vi "Load Budget.vi"(8 "error in (no error)":errorcluster, 11 "Budgetizer in":refnum<class "Budgetizer.lvclass">) -> (0 "error out":errorcluster, 3 "Budgetizer out":refnum<class "Budgetizer.lvclass">)   [LabVIEW 2018, in "Budgetizer.lvclass"]
uses:
  Budgetizer.lvclass
  Budgetizer.lvclass/Budgetizer.ctl
  database/Database.lvclass
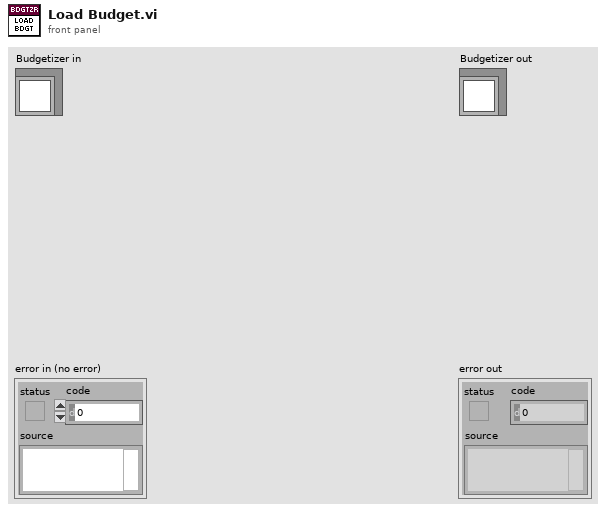
[diagram p1: front panel]
types:
  T1 = enum16{"January", "February", "March", "April", "May", "June", "July", "August", "September", "October", "November", "December"}
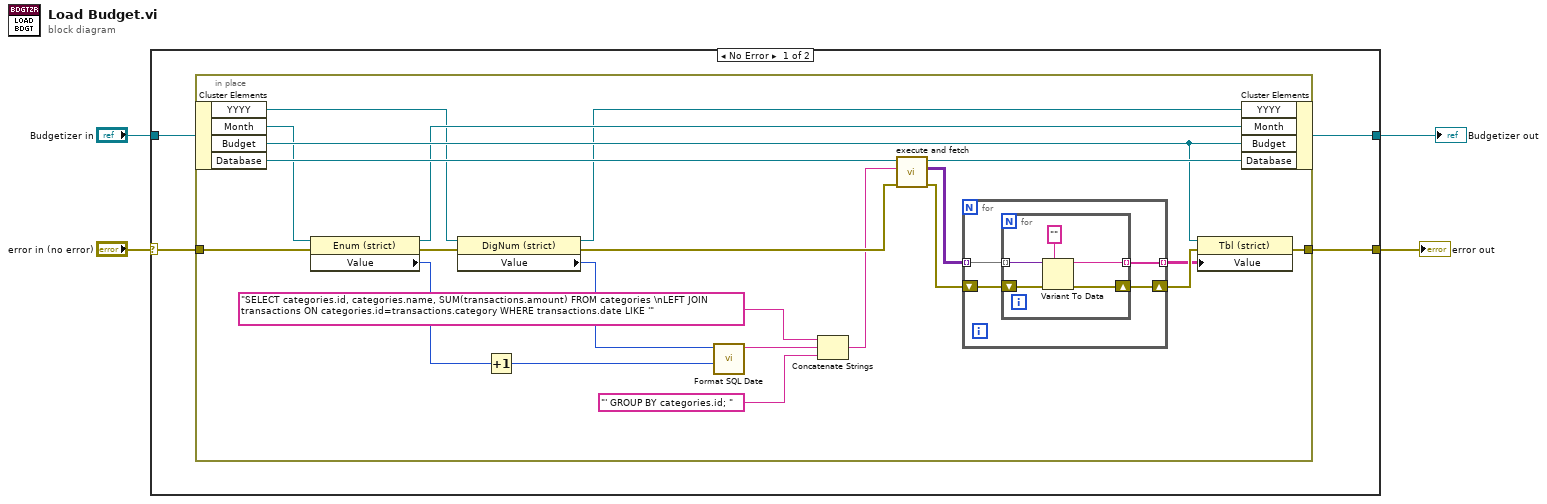
[diagram p0: block diagram]
diagram:
  n1 = case shown="No Error" "error in (no error)" {
    selector: "error in (no error)" -> [w6 w41]
    tunnel: [w5 w41] -> w3
    tunnel: [w7 w40] -> w1
    tunnel: "Budgetizer in" -> [w8 w40]
    frame No Error {
      n2 = in-place {
        in-place-border: w6 -> [w20]
        in-place-border: [w24] -> w5
        n3 = in-place-cluster #1(w8) -> ("YYYY"=w17:refnum<vi>, "Month"=w19:refnum<vi>, "Budget"=w23:refnum<vi>, "Database"=w30:refnum<class "Database.lvclass">)
        n4 = property class="Enum (strict)"(reference=w19, error in=w20) -> (reference out=w18:refnum<vi>, error out=w21:errorcluster, "Value"=w22:T1)
        n5 = property class="DigNum (strict)"(reference=w17, error in=w21) -> (reference out=w16:refnum<vi>, error out=w15:errorcluster, "Value"=w10:i32)
        n6 = Increment(x=w22) -> (x+1=w11:T1)
        n7 = call "Format SQL Date.vi"("Month"=w11, "YYYY"=w10) -> ("YYYY-MM-%"=w14:string)  [unwired: 9 in]
        n8 = Concatenate Strings("SELECT categories.id, categories.name, SUM(transactions.amount) FROM categories \nLEFT JOIN transactions ON categories.id=transactions.category WHERE transactions.date LIKE '", w14, "' GROUP BY categories.id; ") -> (w9:string)
        n9 = call "execute and fetch.vi"("error in (no error)"=w15, "SQL query"=w9, "Database in"=w30) -> ("error out"=w25:errorcluster, "recordset data"=w26:variant[][], "Database out"=w29:refnum<class "Database.lvclass">)  [unwired: 5 in, 1 out]
        n10 = for {
          tunnel: w26 -> [w34] mode=indexing
          shift-right: [w32] -> w28
          shift-left: w25 -> [w33]
          tunnel: [w31] -> w27 mode=indexing
          n11 = for {
            tunnel: w34 -> [w39] mode=indexing
            shift-right: [w37] -> w32
            shift-left: w33 -> [w38]
            tunnel: [w35] -> w31 mode=indexing
            n12 = Variant To Data(error in=w38, type="", Variant=w39) -> (data=w35:string, error out=w37:errorcluster)
          }
        }
        n13 = property class="Tbl (strict)"(reference=w23, error in=w28, "Value"=w27) -> (error out=w24:errorcluster)  [unwired: 1 out]
        n14 = in-place-cluster #1("YYYY"=w16, "Month"=w18, "Budget"=w23, "Database"=w29) -> (w7:refnum<class "Budgetizer.lvclass">)
      }
    }
    frame Error {
    }
  }
  "error out" <- w3
  "Budgetizer out" <- w1
